vi "SVR.vi"(8 "error in":errorcluster) -> (0 "error out":errorcluster, 3 "out":refnum<class "SVR.lvclass">)   [LabVIEW 2020]
doc: "Epsilon-Support Vector Regression.\n\n The free parameters in the model are C and epsilon.\n\n The implementation is based on libsvm. The fit time complexity\n is more than quadratic with the number of samples which makes it hard\n to scale to datasets with more than a couple of 10000 samples. For large\n datasets consider using :class:`~sklearn.svm.LinearSVR` or\n :class:`~sklearn.linear_model.SGDRegressor` instead, possibly after a\n :class:`~sklearn.kernel_approximation.Nystroem` transformer.\n\n Read more in the :ref:`User Guide <svm_regression>`.\n\n Parameters\n ----------\n kernel : {'linear', 'poly', 'rbf', 'sigmoid', 'precomputed'}, default='rbf'\n Specifies the kernel type to be used in the algorithm.\n It must be one of 'linear', 'poly', 'rbf', 'sigmoid', 'precomputed' or\n a callable.\n If none is given, 'rbf' will be used. If a callable is given it is\n used to precompute the kernel matrix.\n\n degree : int, default=3\n Degree of the polynomial kernel function ('poly').\n Ignored by all other kernels.\n\n gamma : {'scale', 'auto'} or float, default='scale'\n Kernel coefficient for 'rbf', 'poly' and 'sigmoid'.\n\n - if ``gamma='scale'`` (default) is passed then it uses\n 1 / (n_features * X.var()) as value of gamma,\n - if 'auto', uses 1 / n_features.\n\n .. versionchanged:: 0.22\n The default value of ``gamma`` changed from 'auto' to 'scale'.\n\n coef0 : float, default=0.0\n Independent term in kernel function.\n It is only significant in 'poly' and 'sigmoid'.\n\n tol : float, default=1e-3\n Tolerance for stopping criterion.\n\n C : float, default=1.0\n Regularization parameter. The strength of the regularization is\n inversely proportional to C. Must be strictly positive.\n The penalty is a squared l2 penalty.\n\n epsilon : float, default=0.1\n Epsilon in the epsilon-SVR model. It specifies the epsilon-tube\n within which no penalty is associated in the training loss function\n with points predicted within a distance epsilon from the actual\n value.\n\n shrinking : bool, default=True\n Whether to use the shrinking heuristic.\n See the :ref:`User Guide <shrinking_svm>`.\n\n cache_size : float, default=200\n Specify the size of the kernel cache (in MB).\n\n verbose : bool, default=False\n Enable verbose output. Note that this setting takes advantage of a\n per-process runtime setting in libsvm that, if enabled, may not work\n properly in a multithreaded context.\n\n max_iter : int, default=-1\n Hard limit on iterations within solver, or -1 for no limit.\n\n Attributes\n ----------\n class_weight_ : ndarray of shape (n_classes,)\n Multipliers of parameter C for each class.\n Computed based on the ``class_weight`` parameter.\n\n coef_ : ndarray of shape (1, n_features)\n Weights assigned to the features (coefficients in the primal\n problem). This is only available in the case of a linear kernel.\n\n `coef_` is readonly property derived from `dual_coef_` and\n `support_vectors_`.\n\n dual_coef_ : ndarray of shape (1, n_SV)\n Coefficients of the support vector in the decision function.\n\n fit_status_ : int\n 0 if correctly fitted, 1 otherwise (will raise warning)\n\n intercept_ : ndarray of shape (1,)\n Constants in decision function.\n\n n_support_ : ndarray of shape (n_classes,), dtype=int32\n Number of support vectors for each class.\n\n shape_fit_ : tuple of int of shape (n_dimensions_of_X,)\n Array dimensions of training vector ``X``.\n\n support_ : ndarray of shape (n_SV,)\n Indices of support vectors.\n\n support_vectors_ : ndarray of shape (n_SV, n_features)\n Support vectors.\n\n \nAvailable methods:\nFit\nPredict\nScore\nGet Attributes\nGet Params\nSet Params"
uses:
  SVR.lvclass
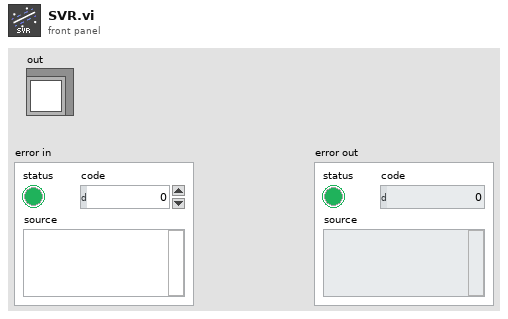
[diagram p1: front panel]
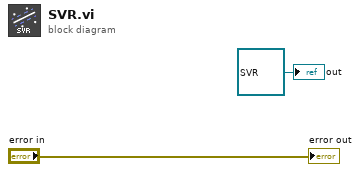
[diagram p0: block diagram]
diagram:
  "out" <- refnum<class "SVR.lvclass"> refnum ("model")
  "error out" <- "error in"
